vi "Read from Connection.vi"(8 "error in (no error)":errorcluster, 10 "Connection":refnum<class "IConnection.lvclass">, 11 "IMessagingProtocol in":refnum<class "IMessagingProtocol.lvclass">) -> (0 "error out":errorcluster, 2 "Data Read":string, 3 "IMessagingProtocol out":refnum<class "IMessagingProtocol.lvclass">)   [LabVIEW 2019, in "Network Interface.lvlib" / "IMessagingProtocol.lvclass"]
uses:
  <vilib>/gpm_packages/@cs/Network-Sink/Source/Network Interface/IMessagingProtocol/IMessagingProtocol.lvclass
  <vilib>/gpm_packages/@cs/Network-Sink/Source/Network Interface/IConnection/IConnection.lvclass
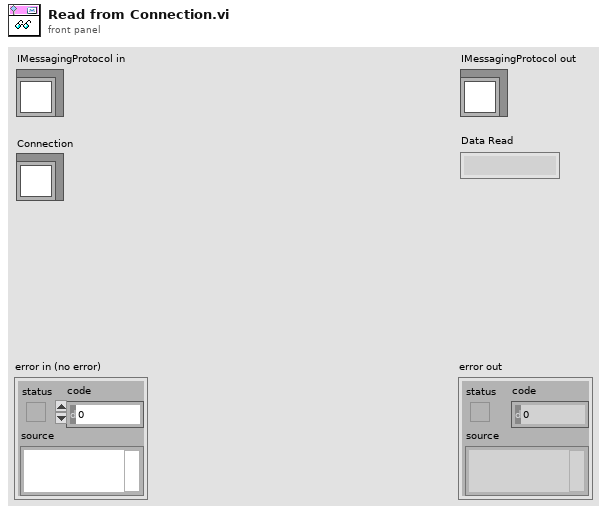
[diagram p1: front panel]
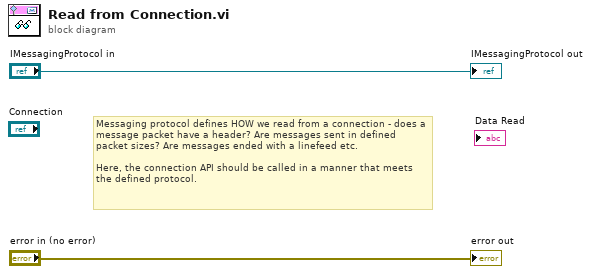
[diagram p0: block diagram]
diagram:
  # "Messaging protocol defines HOW we read from a connection - does a message packet have a header? Are messages sent in defined packet sizes? Are messages ended with a linefeed etc. \n\nHere, the connection API should be called in a manner that meets the defined protocol."
  "error out" <- "error in (no error)"
  "IMessagingProtocol out" <- "IMessagingProtocol in"
